vi "Measure_C_F.vi"(5 "Junction Name":string, 6 "UiDefinition":T1, 7 ".NET Refnum":refnum<k24>, 8 "new file path (Not A Path if cancelled)":path, 10 "appended path":path, 11 ".NET Refnum in":refnum<k24>) -> (0 "error out":errorcluster, 3 "Cluster":cluster{dbl[], dbl[]})   [LabVIEW 2020]
uses:
  UIReferences.ctl
  D:/LabviewDXFViewer/LabviewDXFViewer/bin/Release/LabviewDXFViewer.exe
  LabviewDXFViewer/bin/Release/LabviewDXFViewer.exe
  <vilib>/Analysis/6fits.llb/Curve Fitting Criteria.ctl
  <vilib>/Utility/file.llb/Write Delimited Spreadsheet (DBL).vi
  <vilib>/Utility/file.llb/Write Delimited Spreadsheet (string).vi
  <vilib>/Analysis/NI_AALPro.lvlib
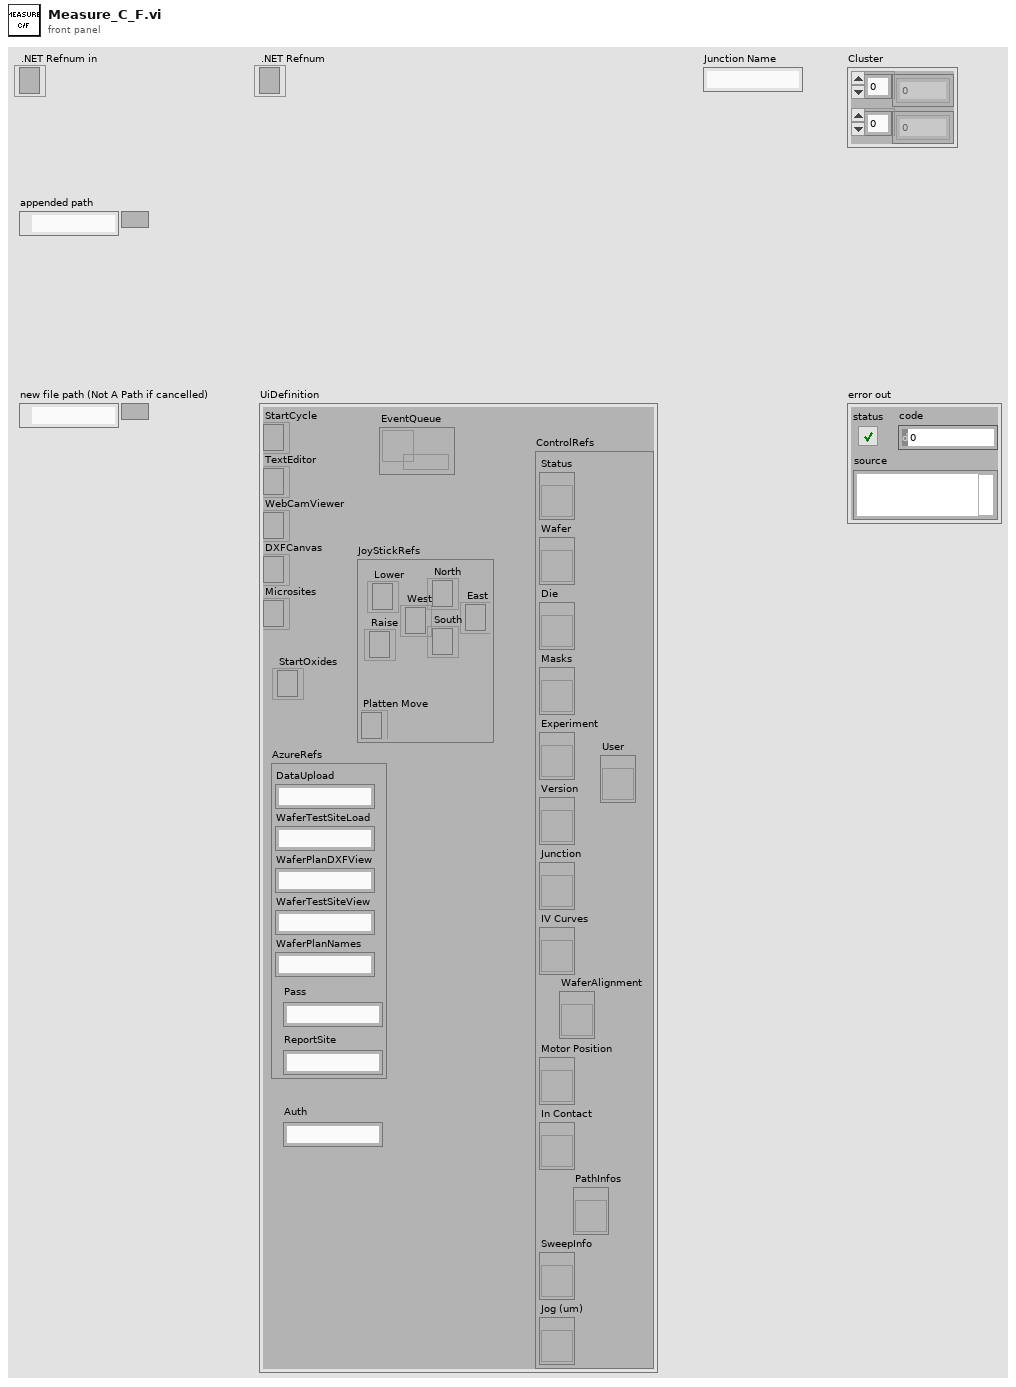
[diagram p1: front panel]
types:
  T1 = typedef "UIReferences.ctl" = cluster{"StartCycle":refnum<k24>, "TextEditor":refnum<k24>, "WebCamViewer":refnum<k24>, "DXFCanvas":refnum<k24>, "Microsites":refnum<k24>, "JoyStickRefs":cluster{"North":refnum<k24>, "Lower":refnum<k24>, "Raise":refnum<k24>, "Platten Move":refnum<k24>, "West":refnum<k24>, "East":refnum<k24>, "South":refnum<k24>}, "AzureRefs":cluster{"DataUpload":string, "WaferTestSiteLoad":string, "WaferPlanDXFView":string, "WaferTestSiteView":string, "WaferPlanNames":string, "Pass":string, "ReportSite":string}, "ControlRefs":cluster{"Status":refnum<vi>, "Wafer":refnum<vi>, "Die":refnum<vi>, "Masks":refnum<vi>, "Experiment":refnum<vi>, "Version":refnum<vi>, "Junction":refnum<vi>, "IV Curves":refnum<vi>, "Motor Position":refnum<vi>, "In Contact":refnum<vi>, "SweepInfo":refnum<vi>, "Jog (um)":refnum<vi>, "PathInfos":refnum<vi>, "User":refnum<vi>, "WaferAlignment":refnum<vi>}, "EventQueue":refnum<queue>, "StartOxides":refnum<k24>, "Auth":string}
  T2 = typedef "NI_AALPro.lvlib/Curve Fitting Criteria.ctl" = u16
  T3 = typedef "CapacitanceInfos.ctl" = cluster{"Conductance":dbl, "CapacitanceIV":dbl, "Intercept":dbl, "CapacitanceSW":dbl, "Sum":dbl, "CapacitanceInfos":T4[], "CapacitancePhase":dbl, "dC/dV":dbl, "Function":string, "OtherInfo":dbl[][], "ChargeCapacitance":dbl, "FitCurves":dbl[][], "Error":dbl, "bestFit":cluster{"Conductance":dbl, "Current0":dbl, "AmpCharge":dbl, "ChargeRC":dbl, "V0":dbl}}
  T4 = typedef "CapacitanceRecord.ctl" = cluster{"Freq":dbl, "Vpp":dbl, "PhaseS":dbl, "Irms":dbl, "PhaseC":dbl, "Theta":dbl, "VDrive":dbl, "Capacitance":dbl, "Other":dbl}
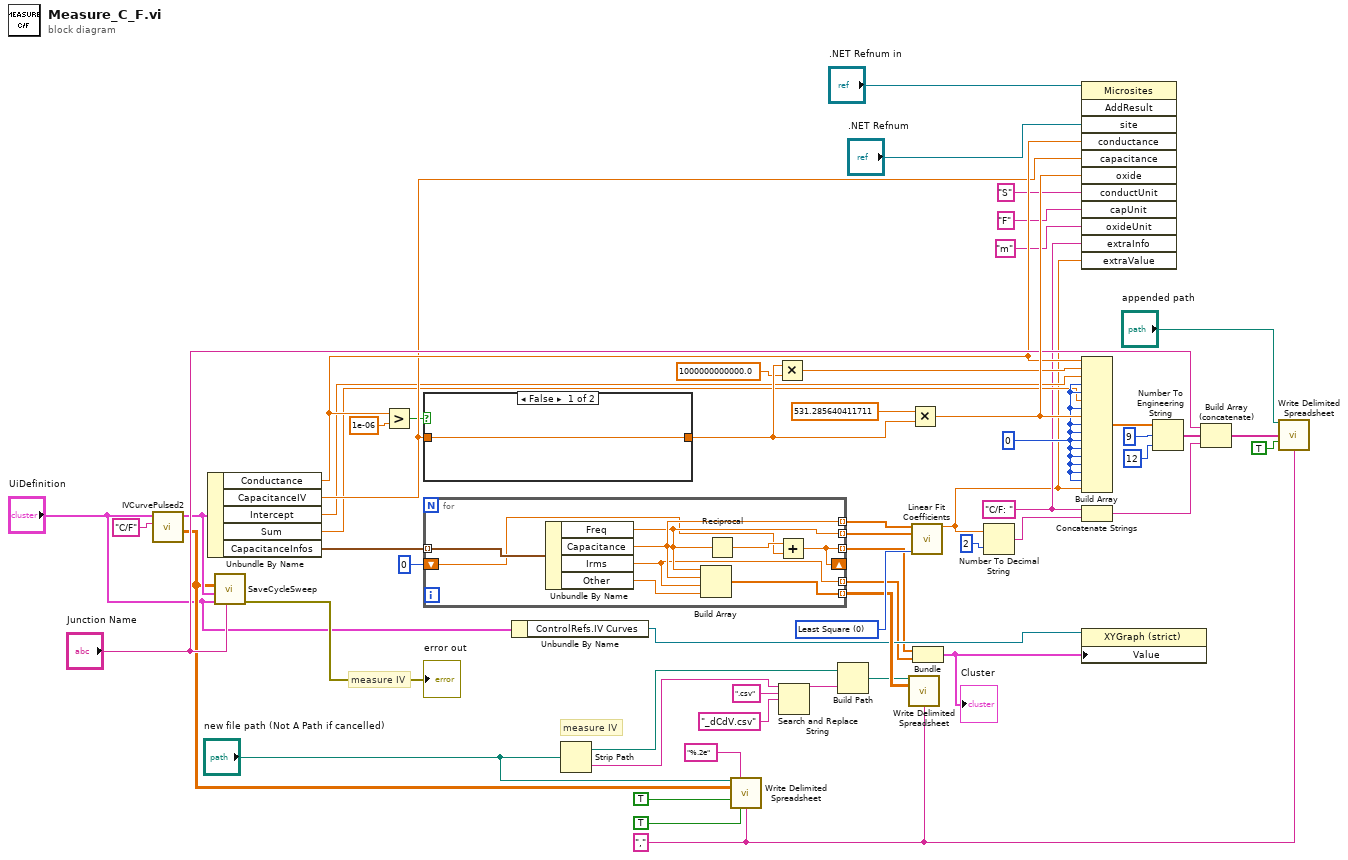
[diagram p0: block diagram]
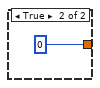
[diagram p2: hidden frame]
diagram:
  w2 = "C/F: "
  w12 = "," ("delimiter (\\t)")
  w50 = T2 0 items=["Least Square", "Least Absolute Residual", "Bisquare"] ("method")
  w51 = 0
  # "measure IV"
  # "measure IV"
  n1 = call "IVCurvePulsed2.vi"("Program"="C/F", "UiDefinition"="UiDefinition") -> ("appended array"=w29:dbl[][], "InfoCluster"=w42:T3)  [unwired: 8 in]
  n2 = Unbundle By Name(w42) -> ("Conductance"=w44:dbl, "CapacitanceIV"=w43:dbl, "Intercept"=w32:dbl, "Sum"=w33:dbl, "CapacitanceInfos"=w45:T4[])
  n3 = call "SaveCycleSweep.vi"("JunctionName"="Junction Name", "UiDefinition 2"="UiDefinition", "InfoCluster"=w42, "appended array"=w29) -> ("error out"=→"error out":errorcluster)  [unwired: 7 in]
  n4 = Greater?(x=w44, y=1e-06) -> (0:w36:bool)
  n5 = case shown="False" w36 {
    tunnel: [w57 0] -> w55
    tunnel: w43 -> [w57 _]
    frame False {
    }
    frame True {
    }
  }
  n6 = for {
    tunnel: w45 -> [w67] mode=indexing
    tunnel: [w64] -> w53 mode=indexing
    tunnel: [w66] -> w52 mode=indexing
    tunnel: [w65] -> w15 mode=indexing
    shift-right: [w61] -> _
    shift-left: 0 -> [w62]
    tunnel: [w61] -> w6 mode=indexing
    tunnel: [w60] -> w7 mode=indexing
    n7 = Unbundle By Name(w67) -> ("Freq"=w64:dbl, "Capacitance"=w66:dbl, "Irms"=w60:dbl, "Other"=w59:dbl)
    n8 = Build Array(w64, w66, w60, w59) -> (w65:dbl[])
    n9 = Reciprocal(x=w64) -> (1/x=w63:dbl)
    n10 = Add(x=w63, y=w62) -> (x+y=w61:dbl)
  }
  n11 = Unbundle By Name("UiDefinition") -> ("ControlRefs.IV Curves"=w10:refnum<vi>)
  n12 = Strip Path(path="new file path (Not A Path if cancelled)") -> (stripped path=w16:path, name=w20:string)
  n13 = call-poly <vilib>:"Write Delimited Spreadsheet.vi"("file path (dialog if empty)"="new file path (Not A Path if cancelled)", "format (%.3f)"="%.2e", "2D data"=w29, "append to file? (new file:F)"=TRUE, "transpose? (no:F)"=TRUE, "delimiter (\\t)"=w12) -> ()  [unwired: 8 in, 2 out]
  n14 = Multiply(x=w55, y=1000000000000.0) -> (x*y=w34:dbl)
  n15 = Search and Replace String(input string=w20, search string=".csv", replace string="_dCdV.csv" ("replace string (\"\")")) -> (result string=w17:string)  [unwired: 5 in, 3 out]
  n16 = Build Path(base path=w16, name or relative path=w17) -> (appended path=w13:path)
  n17 = call-poly <vilib>:"Write Delimited Spreadsheet.vi"("file path (dialog if empty)"=w13, "2D data"=w15, "delimiter (\\t)"=w12) -> ()  [unwired: 11 in, 2 out]
  n18 = Multiply(x=531.285640411711, y=w55) -> (x*y=w56:dbl)
  n19 = call <vilib>:"Linear Fit Coefficients.vi"("Y"=w52, "X"=w53, "method"=w50) -> ("slope"=w1:dbl)  [unwired: 10 in, 2 out]
  n20 = Bundle(w6, w7) -> (w9:cluster{dbl[], dbl[]})  [unwired: 1 in]
  "Cluster" <- w9
  n21 = Number To Decimal String(number=w1, width (-)=i16 2) -> (decimal integer string=w5:string)
  n22 = invoke class="Microsites" method="AddResult"(reference=".NET Refnum in", "site"=".NET Refnum", "conductance"=w44, "capacitance"=w43, "oxide"=w56, "conductUnit"="S", "capUnit"="F", "oxideUnit"="m" ("interceptUnit"), "extraInfo"=w2, "extraValue"=w1) -> ()  [unwired: 2 in, 12 out]
  n23 = Build Array(w44, w34, w32, w51, w51, w33, w51, w56, w51, w51, w51, w51, w51, w51, w51, w51, w1) -> (w31:dbl[])
  n24 = Concatenate Strings(w2, w5) -> (w3:string)
  n25 = property class="XYGraph (strict)"(reference=w10, "Value"=w9) -> ()  [unwired: 1 in, 2 out]
  n26 = Number To Engineering String(2:i16 12 ("precision (6)"), 3:i16 9 ("width (-)"), 4:w31) -> (0:w23:string[])  [unwired: 1 in]
  n27 = Build Array (concatenate)("Junction Name", w23, w3) -> (w25:string[])
  n28 = call-poly <vilib>:"Write Delimited Spreadsheet.vi"("file path (dialog if empty)"="appended path", "1D data"=w25, "append to file? (new file:F)"=TRUE, "delimiter (\\t)"=w12) -> ()  [unwired: 10 in, 2 out]
